vi "IsError.vi"(4 "Error in":errorcluster) -> (1 "Error?":bool)   [LabVIEW 2017, in "GPError.lvlib"]
doc: "<B>Error?</B> will be True only if <B>Error in</B> contains an error.\n\nThis VI supports appended errors, and <B>Error?</B> will be True if just a single one of those is an error.\n\nThis VI is inlined.\n\nSteen Schmidt\nGPower\n14/11 2014"
uses:
  GPError.lvlib
panel:
  # "Copyright © 2014\nGPower\nSee enclosed license file for terms and conditions"
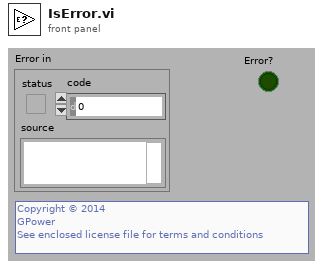
[diagram p1: front panel]
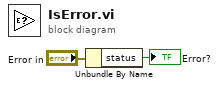
[diagram p0: block diagram]
diagram:
  n1 = Unbundle By Name("Error in") -> ("status"=→"Error?":bool)
